vi "Filter Disconnect Waveforms.vi"(8 "error in (no error)":errorcluster, 11 "Waveform array in":waveform(dbl)[](array[waveform])) -> (0 "error out":errorcluster, 3 "Waveform array out":waveform(dbl)[](array[waveform]))   [LabVIEW 2018, in "TDMS Log.lvlib"]
uses:
  TDMS Log.lvlib
  support/Support Library.lvlib
panel:
  out "Channel Names":string[](array[string])
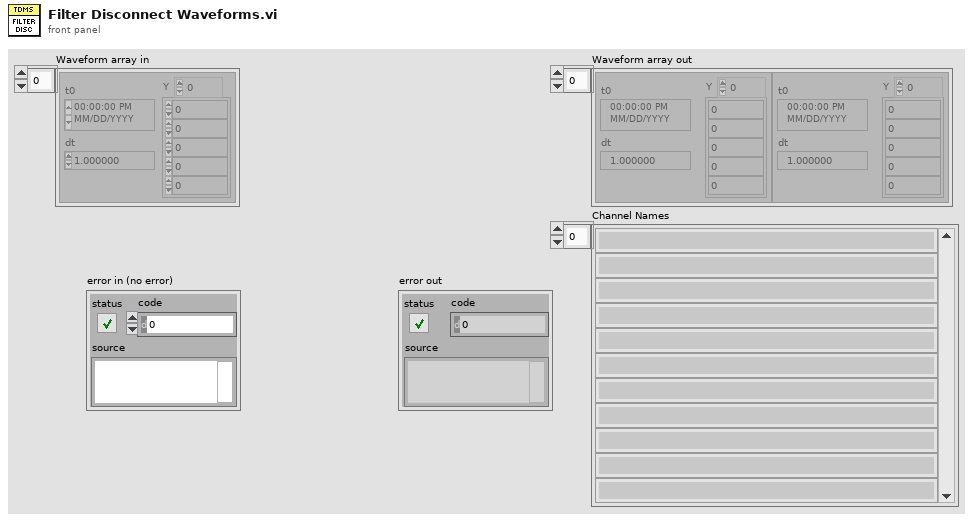
[diagram p1: front panel]
types:
  T1 = cluster{"name":string, "Waveform":waveform(dbl)}[]
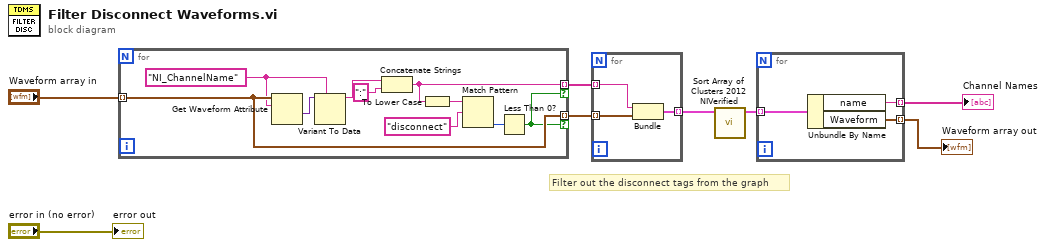
[diagram p0: block diagram]
diagram:
  # "Filter out the disconnect tags from the graph"
  n1 = for {
    tunnel: "Waveform array in" -> [w18] mode=indexing
    tunnel: [w18] -> w5 mode=indexing if=w12
    tunnel: [w9] -> w6 mode=indexing if=w12
    w16 = "NI_ChannelName" ("name")
    n2 = Get Waveform Attribute(6:w16, 7:w18) -> (1:w17:variant)  [unwired: 2 in, 3 out]
    n3 = Variant To Data(type=w16, Variant=w17) -> (data=w10:string)  [unwired: 1 in, 1 out]
    n4 = Concatenate Strings(w10, ":" ("string")) -> (w9:string)
    n5 = To Lower Case(string=w9) -> (all lower case string=w15:string)
    n6 = Match Pattern(string=w15, regular expression="disconnect" ("name")) -> (offset past match=w13:i32)  [unwired: 1 in, 3 out]
    n7 = Less Than 0?(x=w13) -> (x < 0?=w12:bool)
  }
  n8 = for {
    tunnel: w6 -> [w21] mode=indexing
    tunnel: w5 -> [w20] mode=indexing
    tunnel: [w19] -> w4 mode=indexing
    n9 = Bundle(w21, "Waveform"=w20) -> (w19:cluster{string, "Waveform":waveform(dbl)})  [unwired: 1 in]
  }
  n10 = call "Sort Array of Clusters 2012 NIVerified.vi"("Unsorted Array"=w4) -> ("Sorted Array"=w3:T1)  [unwired: 10 in]
  n11 = for {
    tunnel: w3 -> [w24] mode=indexing
    tunnel: [w23] -> w2 mode=indexing
    tunnel: [w22] -> w1 mode=indexing
    n12 = Unbundle By Name(w24) -> ("name"=w23:string, "Waveform"=w22:waveform(dbl))
  }
  "Waveform array out" <- w1
  "Channel Names" <- w2
  "error out" <- "error in (no error)"
